vi "Write movement.vi"(8 "error in (no error)":errorcluster, 10 "movement":string, 11 "BabyHuman in":refnum<class "BabyHuman.lvclass">) -> (0 "error out":errorcluster, 3 "BabyHuman out":refnum<class "BabyHuman.lvclass">)   [LabVIEW 2017, in "BabyHuman.lvclass"]
uses:
  BabyHuman.lvclass
  BabyHuman.lvclass/BabyHuman.ctl
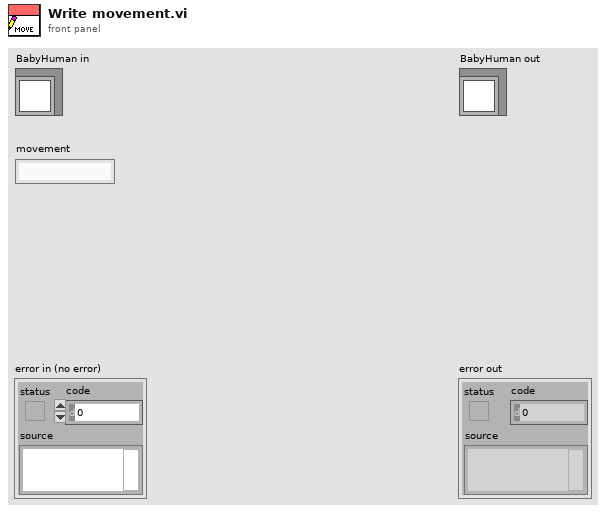
[diagram p1: front panel]
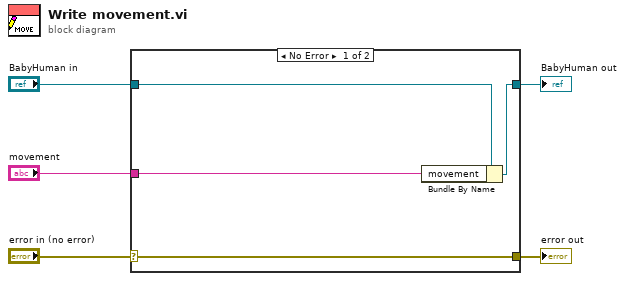
[diagram p0: block diagram]
diagram:
  n1 = case shown="No Error" "error in (no error)" {
    selector: "error in (no error)" -> [w9 w10]
    tunnel: [w9 w10] -> w4
    tunnel: [w7 w11] -> w2
    tunnel: "BabyHuman in" -> [w8 w11]
    tunnel: "movement" -> [w6 _]
    frame No Error {
      n2 = Bundle By Name(cluster=w8, "movement"=w6) -> (w7:refnum<class "BabyHuman.lvclass">)
    }
    frame Error {
    }
  }
  "error out" <- w4
  "BabyHuman out" <- w2
